vi "collectCI1_tt.vi"() -> (1 "size(s)":i32)   [LabVIEW 2013]
uses:
  <vilib>/DAQmx/read.llb/DAQmx Read (Counter 1D U32 1Chan NSamp).vi
  <vilib>/DAQmx/miscellaneous.llb/DAQmx Fill In Error Info.vi
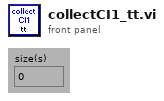
[diagram p1: front panel]
types:
  T1 = typedef "LVRectTypeDef.ctl" = cluster{"Left":i16, "Top":i16, "Right":i16, "Bottom":i16}
  T2 = cluster{"Xpixels":i32, "Vxminref":dbl, "Vxmaxref":dbl, "P":dbl, "Ypixels":i32, "Vyminref":dbl, "Vymaxref":dbl, "srate":sgl, "sAOxy":i32, "timeout":dbl, "type":string, "date":string, "time":string, "Colormap":u16, "Drawing Mode":u16, "Scanning Mode":u16, "square pixels":bool, "square matrix":bool, "Xpixels Img":i32, "Vx-min Img":dbl, "VX-max Img":dbl, "Ypixels Img":i32, "Vy-min Img":dbl, "Vy-max Img ":dbl, "Angle Img":dbl, "autoshutter":bool, "finite":bool, "cont":bool, "wavdet":bool, "measpoints":i32, "avpp":i32, "bufferAO":i32, "bufferAI":i32, "CH1":bool, "CH2":bool, "X":bool, "Y":bool, "Ip":bool, "Vp":bool, "starttick":u32, "waveform":path, "Vx-ref":dbl, "Vy-ref":dbl, "refreshrate":dbl, "refreshbuffer":i32, "tt_cycles":i32, "motorref":refnum<k7>, "mirrorswitch":refnum<k7>, "sample mode":i32, "maxbufferAI":i32, "sampletreshold":dbl, "srateAODO":sgl, "bin":sgl, "Pel":sgl, "Angle draw":dbl, "srate Img":sgl, "ROIimg_plotbounds":T1, "auto OD":bool, "ODfilt":u16, "reset AO_DO":bool}
  T3 = cluster{" CI1":refnum<k21>, "E_CI1":errorcluster}
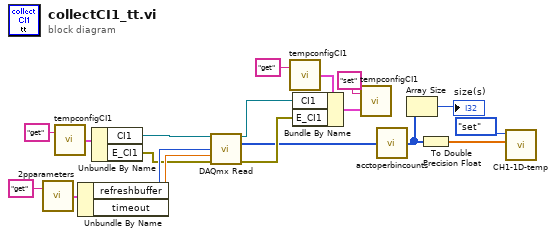
[diagram p0: block diagram]
diagram:
  n1 = call "2pparameters.vi"("command"="get") -> ("Params out"=w17:T2)  [unwired: 1 in]
  n2 = call "tempconfigCI1.vi"("command"="get") -> ("Temp Config out"=w11:T3)  [unwired: 1 in]
  n3 = Unbundle By Name(w17) -> ("refreshbuffer"=w18:i32, "timeout"=w19:dbl)
  n4 = Unbundle By Name(w11) -> ("CI1"=w12:refnum<k21>, "E_CI1"=w13:errorcluster)
  n5 = call-poly <vilib>:"DAQmx Read.vi"("task/channels in"=w12, "number of samples per channel"=w18, "timeout"=w19, "error in"=w13) -> ("task out"=w14:refnum<k21>, "data"=w3:u32[], "error out"=w15:errorcluster)  [unwired: 9 in]
  n6 = call "tempconfigCI1.vi"("command"="get") -> ("Temp Config out"=w9:T3)  [unwired: 1 in]
  n7 = Bundle By Name(cluster=w9, "CI1"=w14, "E_CI1"=w15) -> (w6:T3)
  n8 = call "tempconfigCI1.vi"("Temp Config in"=w6, "command"="set") -> ()  [unwired: 1 out]
  n9 = call "acctoperbincounts.vi"("accumulative counts"=w3) -> ("counts per bin"=w4:u32[])
  n10 = Array Size(array=w4) -> (size(s)=→"size(s)":i32)
  n11 = To Double Precision Float(number=w4) -> (double precision float=w2:dbl[])
  n12 = call "CH1-1D-temp.vi"("array in"=w2, "command"=enum16{"get", "set", "clear", "append"}."set") -> ()  [unwired: 2 in, 2 out]
